vi "Selection.Convert.Set.vi"(8 "error in (no error)":errorcluster, 10 "Selections":T1={"Pull In Time"=FALSE, "Pull In Max Current"=FALSE, "Pull In Max Voltage"=TRUE, "Hold In Time"=FALSE, "Hold In Max Current"=FALSE, "Hold In Min Current"=FALSE, "Hold In Avg Current"=FALSE, "Hold In Avg Max Current"=FALSE, "Hold In Avg Min Current"=FALSE, "Hold In Max Voltage"=FALSE, "Hold In Min Voltage"=FALSE, "Hold In Avg Voltage"=FALSE, "Hold In Avg Max Voltage"=FALSE, "Hold In Avg Min Voltage"=FALSE, "Off Time"=FALSE, "Off Stage Max Current"=FALSE, "Off Stage Min Current"=FALSE, "Off Stage Avg Current"=FALSE, "Total Voltage Pulses"=FALSE, "Total Stage Time"=TRUE}, 11 "ListBox in":refnum<vi>) -> (0 "error out":errorcluster)   [LabVIEW 2015, in "Fuel Injector Analysis Addon System Explorer.lvlib"]
uses:
  Fuel Injector Analysis Addon System Explorer.lvlib
  Shared/Types/Analysis.Channels.Select.ctl
  Shared/Fuel Injector Analysis Addon Shared.lvlib
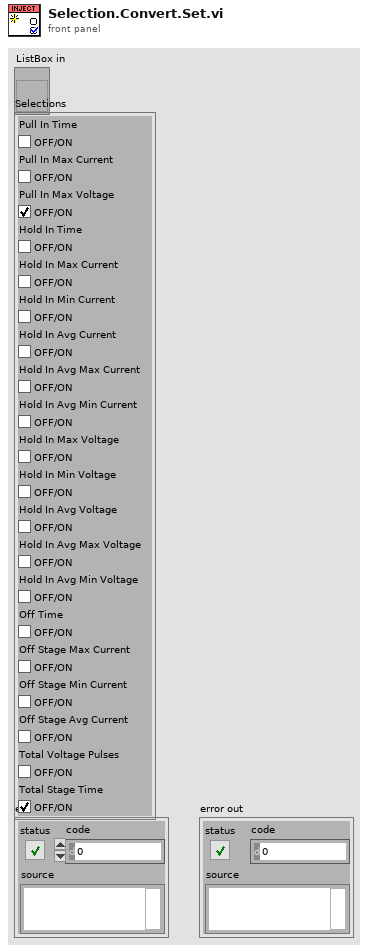
[diagram p1: front panel]
types:
  T1 = typedef "Fuel Injector Analysis Addon Shared.lvlib/Analysis.Channels.Select.ctl" = cluster{"Pull In Time":bool, "Pull In Max Current":bool, "Pull In Max Voltage":bool, "Hold In Time":bool, "Hold In Max Current":bool, "Hold In Min Current":bool, "Hold In Avg Current":bool, "Hold In Avg Max Current":bool, "Hold In Avg Min Current":bool, "Hold In Max Voltage":bool, "Hold In Min Voltage":bool, "Hold In Avg Voltage":bool, "Hold In Avg Max Voltage":bool, "Hold In Avg Min Voltage":bool, "Off Time":bool, "Off Stage Max Current":bool, "Off Stage Min Current":bool, "Off Stage Avg Current":bool, "Total Voltage Pulses":bool, "Total Stage Time":bool}
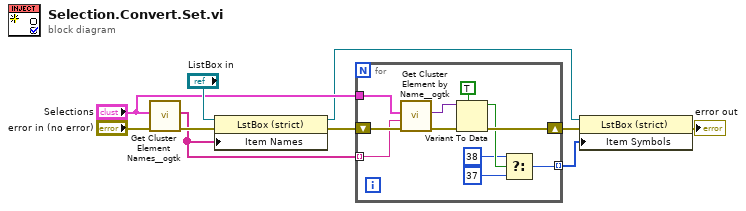
[diagram p0: block diagram]
diagram:
  n1 = call <userlib>:"Get Cluster Element Names__ogtk.vi"("error in (no error)"="error in (no error)", "Cluster"="Selections") -> ("error out"=w6:errorcluster, "Element Names"=w2:string[])  [unwired: 8 in]
  n2 = property class="LstBox (strict)"(reference="ListBox in", error in=w6, "Item Names"=w2) -> (reference out=w5:refnum<vi>, error out=w4:errorcluster)
  n3 = for {
    shift-right: [w16] -> w3
    shift-left: w4 -> [w21]
    tunnel: "Selections" -> [w20]
    tunnel: w2 -> [w19] mode=indexing
    tunnel: [w11] -> w1 mode=indexing
    n4 = call <userlib>:"Get Cluster Element by Name__ogtk.vi"("error in (no error)"=w21, "Element Name"=w19, "Cluster"=w20) -> ("error out"=w18:errorcluster, "VElement"=w17:variant)  [unwired: 6 in, 1 out]
    n5 = Variant To Data(error in=w18, type=TRUE, Variant=w17) -> (data=w14:bool, error out=w16:errorcluster)
    n6 = Select(t=38, s=w14, f=37) -> (s? t:f=w11:i32)
  }
  n7 = property class="LstBox (strict)"(reference=w5, error in=w3, "Item Symbols"=w1) -> (error out=→"error out":errorcluster)  [unwired: 1 out]
